vi "Throttle.vi"(0 "Up":bool, 5 "Down":bool, 7 "X (IN)":dbl, 9 "Y (IN)":dbl, 11 "Rotation (IN)":dbl) -> (6 "Throttle":dbl, 8 "X (OUT)":dbl, 10 "Y (OUT)":dbl, 15 "Rotation (OUT)":dbl)   [LabVIEW 2014]
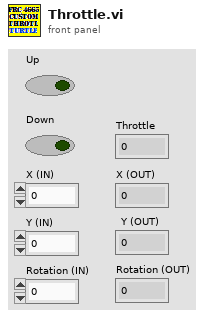
[diagram p1: front panel]
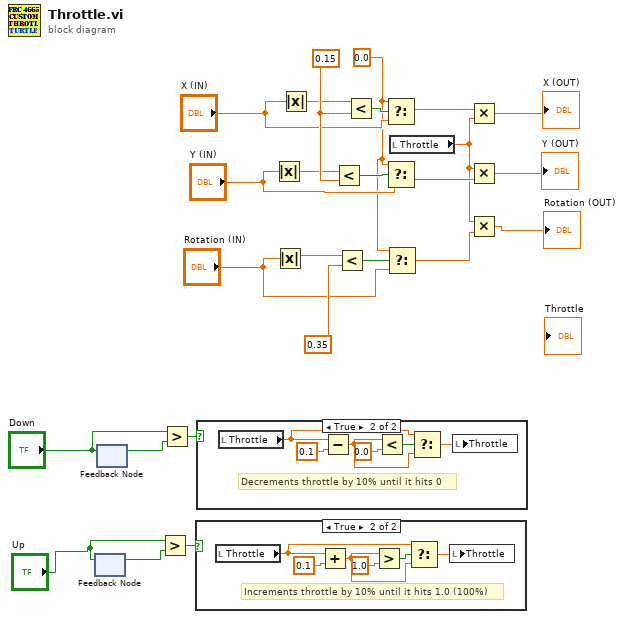
[diagram p0: block diagram]
diagram:
  w2 = 0.0
  w24 = 0.15
  n1 = feedback #1() -> (w13:bool)  [unwired: 1 in]
  n2 = feedback-in #1("Up") -> ()
  n3 = feedback #2() -> (w14:bool)  [unwired: 1 in]
  n4 = feedback-in #2("Down") -> ()
  n5 = Greater?(x="Up", y=w13) -> (0:w12:bool)
  n6 = Greater?(x="Down", y=w14) -> (0:w15:bool)
  n7 = case shown="True" w12 {
    frame False {
    }
    frame True {
      # "Increments throttle by 10% until it hits 1.0 (100%)"
      n8 = local read "Throttle"() -> (w28:dbl)
      n9 = Add(x=w28, y=0.1) -> (x+y=w27:dbl)
      n10 = Greater?(x=w27, y=1.0) -> (0:w29:bool)
      n11 = Select(t=w28, s=w29, f=w27) -> (s? t:f=w26:dbl)
      n12 = local write "Throttle"(w26) -> ()
    }
  }
  n13 = case shown="True" w15 {
    frame False {
    }
    frame True {
      # "Decrements throttle by 10% until it hits 0"
      n14 = local read "Throttle"() -> (w36:dbl)
      n15 = Subtract(x=w36, y=0.1) -> (x-y=w33:dbl)
      n16 = Less?(x=w33, y=0.0) -> (x < y?=w34:bool)
      n17 = Select(t=w36, s=w34, f=w33) -> (s? t:f=w35:dbl)
      n18 = local write "Throttle"(w35) -> ()
    }
  }
  n19 = Absolute Value(x="Y (IN)") -> (abs(x)=w23:dbl)
  n20 = Absolute Value(x="Rotation (IN)") -> (abs(x)=w3:dbl)
  n21 = Absolute Value(x="X (IN)") -> (abs(x)=w22:dbl)
  n22 = Less?(x=w23, y=w24) -> (x < y?=w21:bool)
  n23 = Less?(x=w3, y=0.35) -> (x < y?=w17:bool)
  n24 = Less?(x=w22, y=w24) -> (x < y?=w25:bool)
  n25 = Select(t=w2, s=w25, f="X (IN)") -> (s? t:f=w18:dbl)
  n26 = Select(t=w2, s=w21, f="Y (IN)") -> (s? t:f=w20:dbl)
  n27 = Select(t=w2, s=w17, f="Rotation (IN)") -> (s? t:f=w1:dbl)
  n28 = local read "Throttle"() -> (w19:dbl)
  n29 = Multiply(x=w18, y=w19) -> (x*y=→"X (OUT)":dbl)
  n30 = Multiply(x=w19, y=w20) -> (x*y=→"Y (OUT)":dbl)
  n31 = Multiply(x=w19, y=w1) -> (x*y=→"Rotation (OUT)":dbl)
